vi "Actor Core.vi"(8 "error in":errorcluster, 11 "State in":refnum<class "Sideways Drive.lvclass">) -> (0 "error out":errorcluster, 3 "Actor out":refnum<class "Actor.lvclass">)   [LabVIEW 2014, in "Sideways Drive.lvlib" / "Sideways Drive.lvclass"]
doc: "(<B>Filename</B>: Actor Framework.lvlib:Actor.lvclass:Actor Core.vi)\n\nThis override invokes Entry.vi on the initial state, prior to calling the parent Actor Core. Adding this behavior to Actor Core (instead of an override of Pre Launch Init.vi) allows the initial state to launch a nested actor as part of its entry behavior.\n\nReceives messages to the actor, reacts to them, and initiates any error handling that may shut the actor down.\n\nDescendant classes may override this VI to append parallel tasks for the actor to complete while it handles messages. Overrides use the Call Parent Method node."
uses:
  Sideways Drive.lvclass
  <vilib>/ActorFramework/Actor/Actor.lvclass
  Sideways Drive State.ctl
  Sideways Drive.lvclass/Sideways Drive.ctl
  Motor with Encoders/Motors with Encoders Class/Motors with Encoders.lvclass
  Robot Actor Framework/System Actor/System Actor Class/System Actor.lvclass
panel:
  in  "Sideways Drive State":T1 {"Sideways Drive Power" min=-1.0 max=1.0 scale=-1.0..1.0}
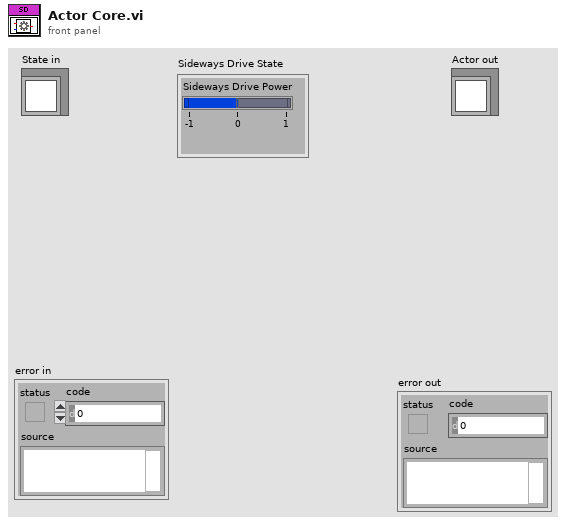
[diagram p1: front panel]
types:
  T1 = typedef "Sideways Drive.lvlib/Sideways Drive.lvclass/Sideways Drive State.ctl" = cluster{"Sideways Drive Power ":dbl}
  T2 = enum16{"Critical", "Error", "Warning", "Informational", "Debug"}
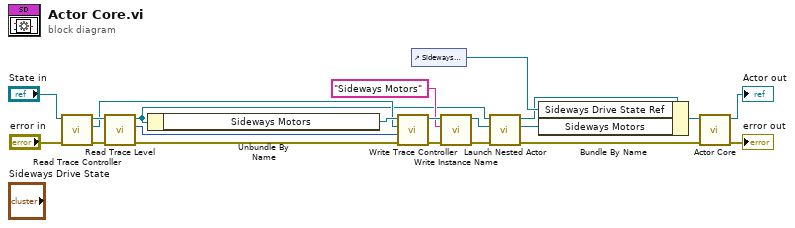
[diagram p0: block diagram]
diagram:
  n1 = call-dynamic "Read Trace Controller.vi"("error in (no error)"="error in", "System Actor in"="State in") -> ("error out"=w7:errorcluster, "Trace Controller"=w14:refnum<class "Message Enqueuer.lvclass">, "System Actor out"=w17:refnum<class "Sideways Drive.lvclass">)  [unwired: 7 in]
  n2 = call-dynamic "Read Trace Level.vi"("error in (no error)"=w7, "System Actor in"=w17) -> ("error out"=w6:errorcluster, "Trace Level"=w13:T2, "System Actor out"=w2:refnum<class "Sideways Drive.lvclass">)  [unwired: 7 in]
  n3 = Unbundle By Name(w2) -> ("Sideways Motors"=w15:refnum<class "Motors with Encoders.lvclass">)
  n4 = call-dynamic "Write Trace Controller.vi"("error in (no error)"=w6, "Trace Level"=w13, "Trace Controller"=w14, "System Actor in"=w15) -> ("error out"=w5:errorcluster, "System Actor out"=w12:refnum<class "Motors with Encoders.lvclass">)  [unwired: 6 in]
  n5 = control-ref of="Sideways Drive State"() -> (w18:refnum<vi>)
  n6 = call-dynamic "Write Instance Name.vi"("error in (no error)"=w5, "Instance Name"="Sideways Motors", "System Actor in"=w12) -> ("error out"=w4:errorcluster, "System Actor out"=w10:refnum<class "Motors with Encoders.lvclass">)  [unwired: 7 in]
  n7 = call <vilib>:"Launch Nested Actor.vi"("error in (no error)"=w4, "Nested Actor"=w10, "Caller Actor in"=w2) -> ("error out"=w3:errorcluster, "Nested Actor's Enqueuer"=w9:refnum<class "Message Enqueuer.lvclass">, "Caller Actor out"=w1:refnum<class "Sideways Drive.lvclass">)  [unwired: 6 in]
  n8 = Bundle By Name(cluster=w1, "Sideways Drive State Ref"=w18, "Sideways Motors"=w9) -> (w19:refnum<class "Sideways Drive.lvclass">)
  n9 = call-parent "Actor Core.vi"("error in"=w3, "State in"=w19) -> ("error out"=→"error out":errorcluster, "Actor out"=→"Actor out":refnum<class "Actor.lvclass">)  [unwired: 8 in]
